vi "Write Log11 emibin record.vi"(0 "refnum in":refnum<file>, 5 "Time":timestamp, 7 "Doubles":dbl[](array[numeric]), 9 "u8":u8[](array[numeric]), 11 "error in":errorcluster) -> (4 "refnum out":refnum<file>, 15 "error out":errorcluster)   [LabVIEW 2011]
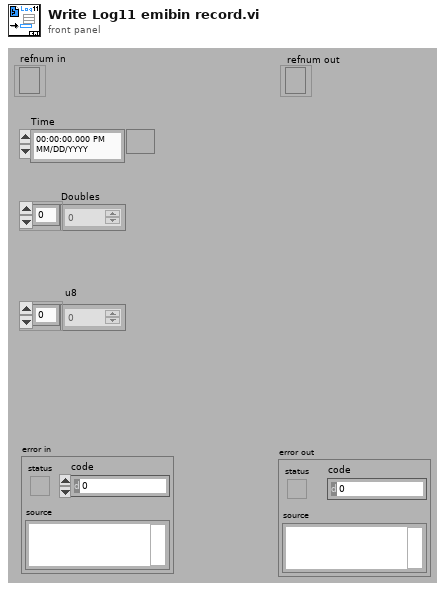
[diagram p1: front panel]
types:
  T1 = enum16{"big-endian, network order", "native, host order", "little-endian"}
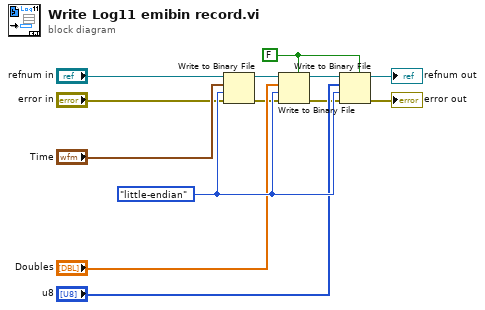
[diagram p0: block diagram]
diagram:
  w13 = T1."little-endian" ("byte order (0:big-endian, network order)")
  w9 = FALSE ("prepend array or string size? (T)")
  n1 = Write to Binary File(file (use dialog)="refnum in", data="Time", error in="error in", 9:w13) -> (refnum out=w2:refnum<file>, error out=w5:errorcluster)  [unwired: 2 in, 1 out]
  n2 = Write to Binary File(file (use dialog)=w2, data="Doubles", error in=w5, 5:w9, 9:w13) -> (refnum out=w1:refnum<file>, error out=w6:errorcluster)  [unwired: 1 in, 1 out]
  n3 = Write to Binary File(file (use dialog)=w1, data="u8", error in=w6, 5:w9, 9:w13) -> (refnum out=→"refnum out":refnum<file>, error out=→"error out":errorcluster)  [unwired: 1 in, 1 out]
